vi "UpdateResultToSFC.vi"(8 "error in":errorcluster, 9 "Message":string, 10 "SN":string, 11 "result":bool) -> (0 "error out":errorcluster)   [LabVIEW 2013]
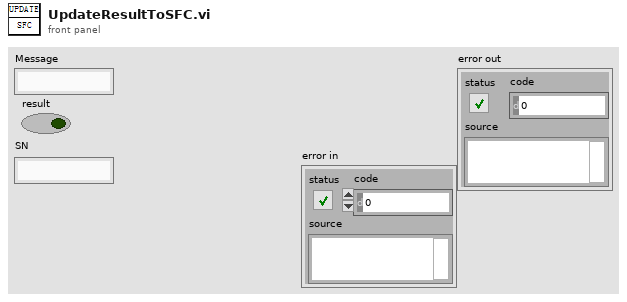
[diagram p1: front panel]
types:
  T1 = enum16{"open", "replace", "create", "open or create", "replace or create", "replace or create with confirmation"}
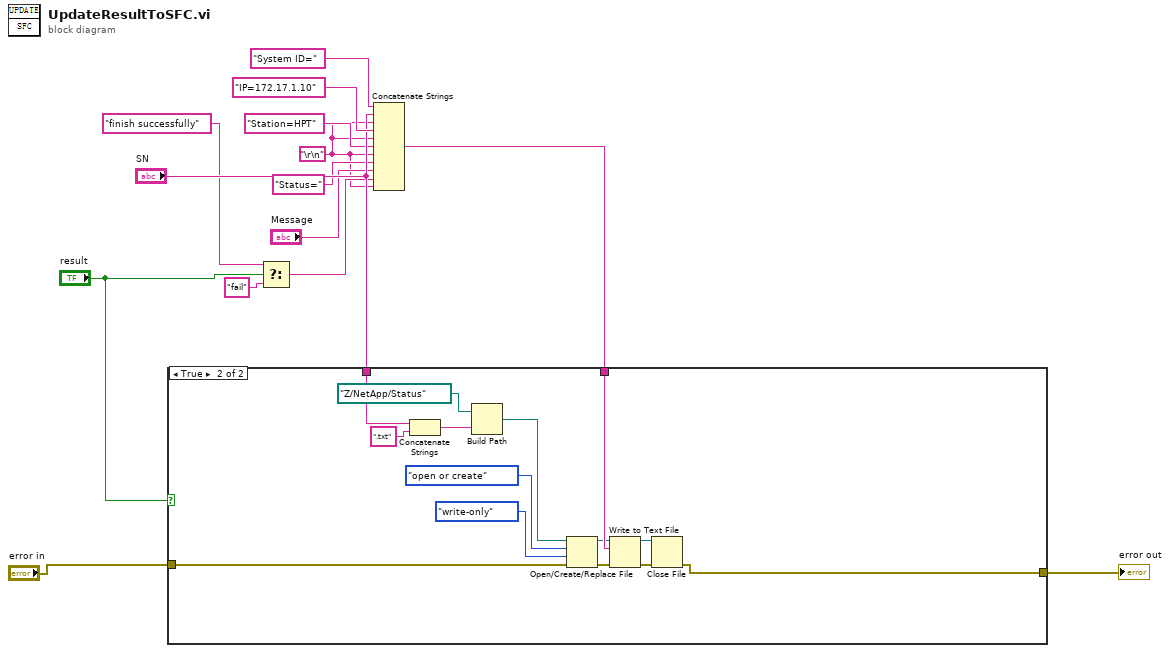
[diagram p0: block diagram]
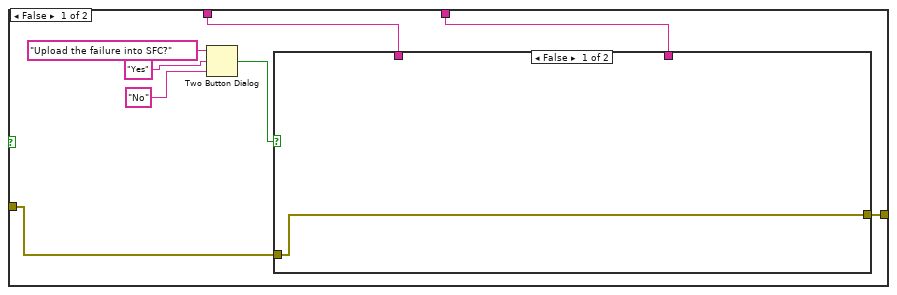
[diagram p2: hidden frame]
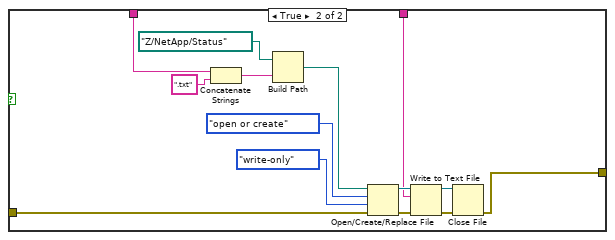
[diagram p3: hidden frame]
diagram:
  w4 = "\r\n"
  n1 = Select(t="finish successfully" ("string"), s="result", f="fail" ("string")) -> (s? t:f=w5:string)
  n2 = Concatenate Strings("System ID=" ("string"), "SN", w4, "IP=172.17.1.10" ("string"), w4, "Station=HPT" ("string"), w4, "Status=" ("string"), "Message", w5, w4) -> (w12:string)
  n3 = case shown="True" "result" {
    tunnel: w12 -> [w17 w46]
    tunnel: "SN" -> [w18 w41]
    tunnel: "error in" -> [w15 w39]
    tunnel: [w16 w38] -> w1
    frame False {
      n4 = Two Button Dialog(message="Upload the failure into SFC?", 1:"No" ("F button name (\"Cancel\")"), 2:"Yes" ("T button name (\"OK\")")) -> (T button?=w19:bool)
      n5 = case shown="False" w19 {
        tunnel: w18 -> [_ w27]
        tunnel: w17 -> [_ w26]
        tunnel: [w23 w25] -> w16
        tunnel: w15 -> [w23 w24]
        frame False {
        }
        frame True {
          n6 = Concatenate Strings(w27, ".txt" ("string")) -> (w28:string)
          n7 = Build Path(base path=path "Z:/NetApp/Status", name or relative path=w28) -> (appended path=w33:path)
          n8 = Open/Create/Replace File(file path (use dialog)=w33, error in=w24, operation (0:open)=T1."open or create", access (0:read/write)=enum16{"read/write", "read-only", "write-only"}."write-only") -> (refnum out=w32:refnum<file>, error out=w31:errorcluster)  [unwired: 2 in, 1 out]
          n9 = Write to Text File(file (use dialog)=w32, text=w26, error in=w31) -> (refnum out=w37:refnum<file>, error out=w36:errorcluster)  [unwired: 1 in, 1 out]
          n10 = Close File(refnum=w37, error in=w36) -> (error out=w25:errorcluster)  [unwired: 1 out]
        }
      }
    }
    frame True {
      n11 = Concatenate Strings(w41, ".txt" ("string")) -> (w40:string)
      n12 = Build Path(base path=path "Z:/NetApp/Status", name or relative path=w40) -> (appended path=w47:path)
      n13 = Open/Create/Replace File(file path (use dialog)=w47, error in=w39, operation (0:open)=T1."open or create", access (0:read/write)=enum16{"read/write", "read-only", "write-only"}."write-only") -> (refnum out=w45:refnum<file>, error out=w44:errorcluster)  [unwired: 2 in, 1 out]
      n14 = Write to Text File(file (use dialog)=w45, text=w46, error in=w44) -> (refnum out=w51:refnum<file>, error out=w50:errorcluster)  [unwired: 1 in, 1 out]
      n15 = Close File(refnum=w51, error in=w50) -> (error out=w38:errorcluster)  [unwired: 1 out]
    }
  }
  "error out" <- w1
